vi "Read PCM CAN ID.vi"(8 "error in (no error)":errorcluster, 11 "Comp Pressure in":refnum<class "Comp Pressure.lvclass">) -> (0 "error out":errorcluster, 2 "PCM CAN ID":u8, 3 "Comp Pressure out":refnum<class "Comp Pressure.lvclass">)   [LabVIEW 2014, in "Comp Pressure.lvlib" / "Comp Pressure.lvclass"]
uses:
  Comp Pressure.lvclass
  Comp Pressure.lvclass/Comp Pressure.ctl
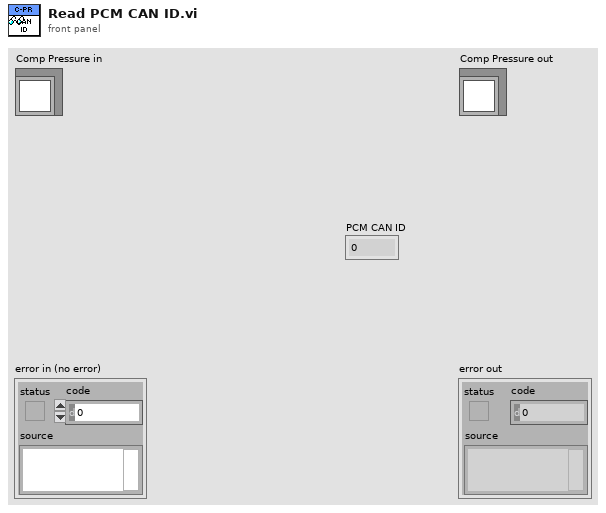
[diagram p1: front panel]
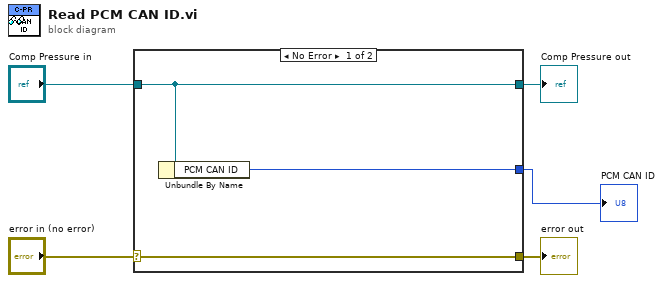
[diagram p0: block diagram]
diagram:
  n1 = case shown="No Error" "error in (no error)" {
    selector: "error in (no error)" -> [w8 w9]
    tunnel: [w8 w9] -> w4
    tunnel: [w7 w10] -> w2
    tunnel: "Comp Pressure in" -> [w7 w10]
    tunnel: [w6 _] -> w1
    frame No Error {
      n2 = Unbundle By Name(w7) -> ("PCM CAN ID"=w6:u8)
    }
    frame Error {
    }
  }
  "error out" <- w4
  "Comp Pressure out" <- w2
  "PCM CAN ID" <- w1
